vi "Append Report Text (num wrap).vi"(0 "report in":refnum<class "NI_report.lvclass">, 1 "MS Office parameters":T1, 2 "format string (%.3f)":string="%.3f", 7 "text":dbl format="%.2f", 9 "append on new line? (F)":bool, 11 "error in (no error)":errorcluster) -> (4 "report out":refnum<class "NI_report.lvclass">, 8 "start out (Word)":i32, 10 "end out (Word)":i32, 15 "error out":errorcluster)   [LabVIEW 2020, in "NI_report.lvclass"]
doc: "Appends text to the selected report. Wire data to the <B>text</B> input to determine the polymorphic instance to use or manually select the instance."
uses:
  <vilib>/Utility/NIReport.llb/NI_report.lvclass
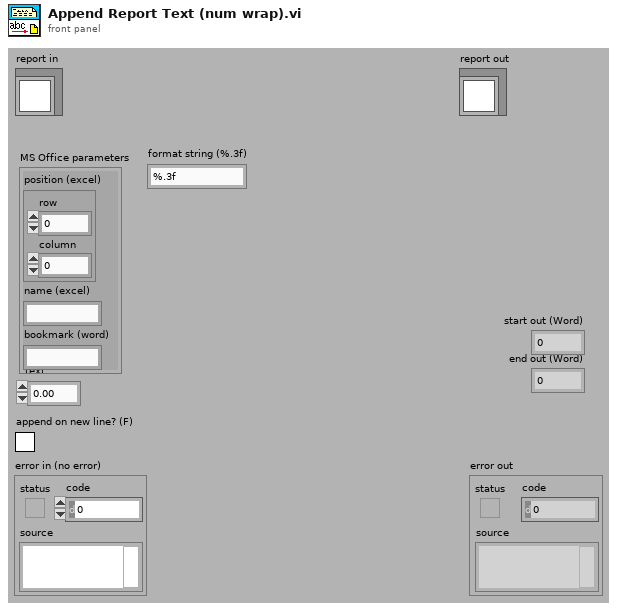
[diagram p1: front panel]
types:
  T1 = cluster{"position (excel)":cluster{"row":i32, "column":i32}, "name (excel)":string, "bookmark (word)":string}
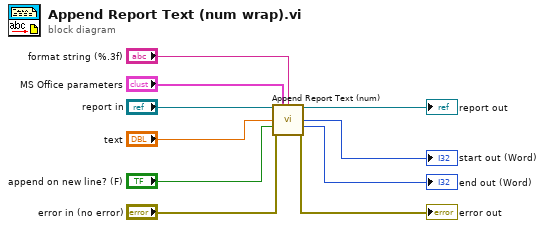
[diagram p0: block diagram]
diagram:
  n1 = call-dynamic "Append Report Text (num).vi"("report in"="report in", "MS Office parameters"="MS Office parameters", "format string (%.3f)"="format string (%.3f)", "text"="text", "append on new line? (F)"="append on new line? (F)", "error in (no error)"="error in (no error)") -> ("report out"=→"report out":refnum<class "NI_report.lvclass">, "start out (Word)"=→"start out (Word)":i32, "end out (Word)"=→"end out (Word)":i32, "error out"=→"error out":errorcluster)  [unwired: 6 out]
